vi "XIPIN_System_Management_Wizard_1_2.vi"   [LabVIEW 2017]
doc: "The System Management Wizard generates an HDL wrapper to configure UltraScale FPGA SYSMON primitive for user-specified channels and alarms.\n------------------------------------\n<b>Need License</b> : No\n<b>Interface</b> : AXI4"
uses:
  <vilib>/rvi/XilinxIP/XIPIN_XNode/niFpgaXIPIN.xnode
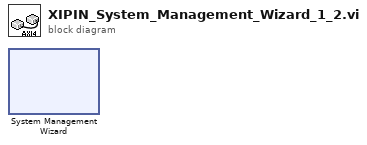
[diagram p0: block diagram]
diagram:
  n1 = xnode ("System Management Wizard")() -> ()
